vi "BeginFlushDrain.vi"(8 "error in (no error)":errorcluster, 10 "managerEnqueuer":refnum<class "Message Enqueuer.lvclass">, 11 "LogManager in":refnum<class "LogManager.lvclass">) -> (0 "error out":errorcluster, 3 "LogManager out":refnum<class "LogManager.lvclass">)   [LabVIEW 2026, in "Lumberjack.lvlib" / "LogManager.lvclass"]
doc: "Start the shutdown flush fence. Seeds the manager's own enqueuer (from managerEnqueuer, provided by Logger.Shutdown via RequestShutdownMsg) into selfEnqueuer, marks the manager as draining, then sends a FlushAppenderMsg (normal priority) to every registered appender so each flushes its sink after draining its statement queue. pendingFlushCount is set to the number of appenders that were successfully sent to; a send that errors (a dead/faulted appender's enqueuer) is skipped and not counted, so shutdown never waits on an ack that cannot come. If no live appender remains (count 0), the manager is sent its own Normal Stop immediately. Community; called by RequestShutdownMsg.Do (SRS-LMBR-002)."
uses:
  LogManager.lvclass
  <vilib>/ActorFramework/Message Enqueuer/Message Enqueuer.lvclass
  LogManager.lvclass/LogManager.ctl
  <vilib>/ActorFramework/Message Enqueuer/Message Enqueuer.lvclass/Message Enqueuer.ctl
  <vilib>/ActorFramework/Message Enqueuer/Enqueue.vi
  <vilib>/ActorFramework/Stop Msg/Stop Msg.lvclass
  C:/Program Files (x86)/National Instruments/LabVIEW 2026/vi.lib/ActorFramework/Message/Message.lvclass
  <vilib>/ActorFramework/Message Priority Queue/Priority Enqueue.vi
  Messages/FlushAppenderMsg.lvclass/FlushAppenderMsg.lvclass
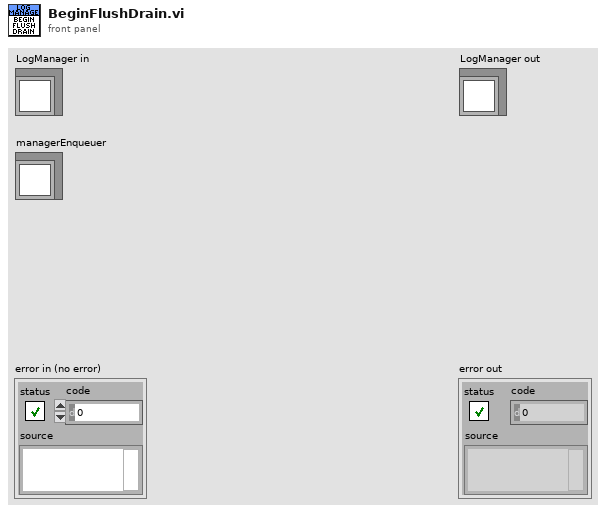
[diagram p1: front panel]
types:
  T1 = typedef "Lumberjack.lvlib/RegistryEntry.ctl" = cluster{"id":string, "enqueuer":refnum<class "Message Enqueuer.lvclass">}
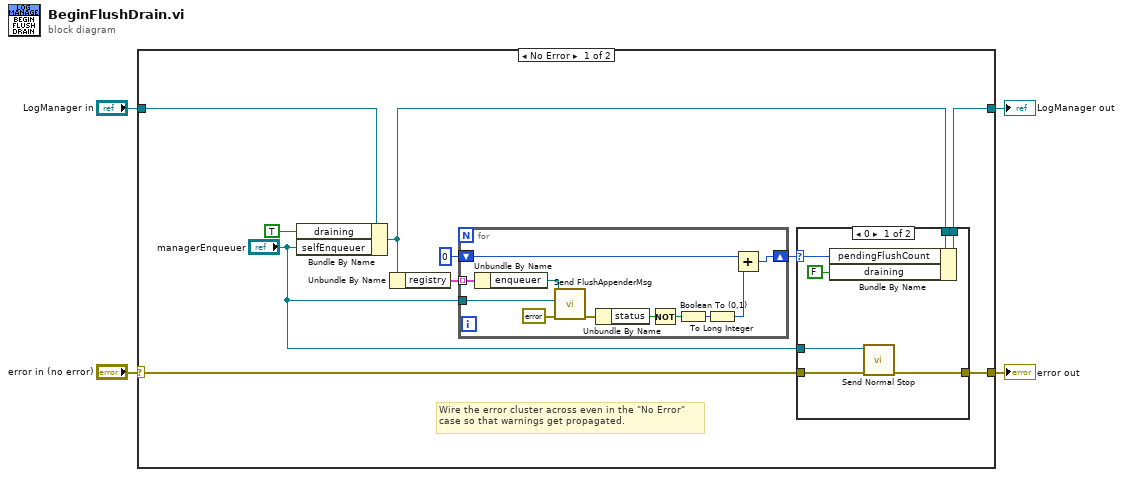
[diagram p0: block diagram]
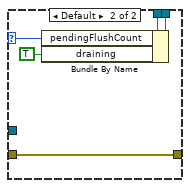
[diagram p2: hidden frame]
diagram:
  n1 = case shown="No Error" "error in (no error)" {
    selector: "error in (no error)" -> [w10 w38]
    tunnel: [w9 w38] -> w3
    tunnel: [w7 w39] -> w1
    tunnel: "LogManager in" -> [w14 w39]
    frame No Error {
      # "Wire the error cluster across even in the \"No Error\"\ncase so that warnings get propagated."
      n2 = Bundle By Name(cluster=w14, "draining"=TRUE, "selfEnqueuer"="managerEnqueuer") -> (w8:refnum<class "LogManager.lvclass">)
      n3 = Unbundle By Name(w8) -> ("registry"=w13:T1[])
      n4 = for {
        tunnel: w13 -> [w37] mode=indexing
        shift-right: [w32] -> w5
        shift-left: 0 -> [w33]
        tunnel: "managerEnqueuer" -> [w35]
        n5 = Unbundle By Name(w37) -> ("enqueuer"=w36:refnum<class "Message Enqueuer.lvclass">)
        n6 = call "Send FlushAppenderMsg.vi"("error in (no error)"=errorcluster {"status"=FALSE, "code"=0, "source"=""}, "replyEnqueuer"=w35, "Enqueuer in"=w36) -> ("error out"=w31:errorcluster)  [unwired: 7 in, 1 out]
        n7 = Unbundle By Name(w31) -> ("status"=w30:bool)
        n8 = Not(x=w30) -> (.not. x?=w29:bool)
        n9 = Boolean To (0,1)(Boolean=w29) -> (0, 1=w28:i16)
        n10 = To Long Integer(number=w28) -> (32bit integer=w27:i32)
        n11 = Add(x=w33, y=w27) -> (x+y=w32:i32)
      }
      n12 = case shown="0" w5 {
        selector: w5 -> [w17 w23]
        tunnel: w10 -> [w21 w26]
        tunnel: [w20 w26] -> w9
        tunnel: w8 -> [w19 w25]
        tunnel: [w18 w24] -> w7
        tunnel: "managerEnqueuer" -> [w15 _]
        frame 0 {
          n13 = Bundle By Name(cluster=w19, "pendingFlushCount"=w17, "draining"=FALSE) -> (w18:refnum<class "LogManager.lvclass">)
          n14 = call <vilib>:"Send Normal Stop.vi"("error in (no error)"=w21, "Message Enqueuer"=w15) -> ("error out"=w20:errorcluster)  [unwired: 9 in]
        }
        frame Default {
          n15 = Bundle By Name(cluster=w25, "pendingFlushCount"=w23, "draining"=TRUE) -> (w24:refnum<class "LogManager.lvclass">)
        }
      }
    }
    frame Error {
    }
  }
  "error out" <- w3
  "LogManager out" <- w1
